vi "Randomize 1D Array.vi"(4 "array":dbl[](array[numeric])) -> (1 "randomized array":dbl[](array[numeric]))   [LabVIEW 2020, in "varilib.lvlib"]
doc: "Returns a randomized version of 1D array."
uses:
  varilib.lvlib
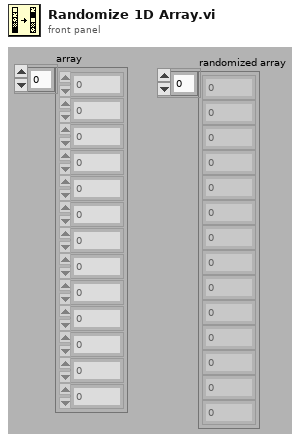
[diagram p1: front panel]
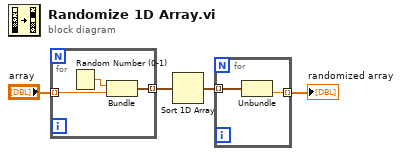
[diagram p0: block diagram]
diagram:
  n1 = for {
    tunnel: "array" -> [w6] mode=indexing
    tunnel: [w5] -> w3 mode=indexing
    n2 = Random Number (0-1)() -> (number: 0 to 1=w7:dbl)
    n3 = Bundle("number: 0 to 1"=w7, w6) -> (w5:cluster{"number: 0 to 1":dbl, dbl})  [unwired: 1 in]
  }
  n4 = Sort 1D Array(array=w3) -> (sorted array=w2:cluster{"number: 0 to 1":dbl, dbl}[])
  n5 = for {
    tunnel: w2 -> [w9] mode=indexing
    tunnel: [w8] -> w1 mode=indexing
    n6 = Unbundle(w9) -> (w8:dbl)  [unwired: 1 out]
  }
  "randomized array" <- w1
